vi "QD Load Debug Snapshot.vi"(6 "Variant in":variant, 7 "Shift Pressed?":bool, 8 "error in (no error)":errorcluster, 10 "QD Combo Box Ref":refnum<vi>, 11 "QD Launch VI Ref":refnum<vi>) -> (0 "error out":errorcluster, 4 "Variant out":variant)   [LabVIEW 2020]
doc: "Restore <b>Debug Snapshot</b> for the current VI. Use SHIFT to ignore breakpoints.\n\nDefault Shortcut - [l]"
uses:
  Public API.lvlib
  Type Definitions/Snapshot Handling Options--cluster.ctl
  Path Getter/Path Getter.lvclass
  C:/Users/juanj/Documents/hasbun_wood_engineering/github/Debug-Snapshots-for-LabVIEW/src/Path Getter/Path Getter.lvclass
  C:/Users/juanj/Documents/hasbun_wood_engineering/github/Debug-Snapshots-for-LabVIEW/src/IPath Getter/IPath Getter.lvclass
panel:
  in  "Undo Name":string="Quick Drop Keyboard Shortcut"
  # "Do not change the connector pane of this VI.\n\nSee the block diagram for directions on how to use this template."
  # "Specify the name of the Undo transaction"
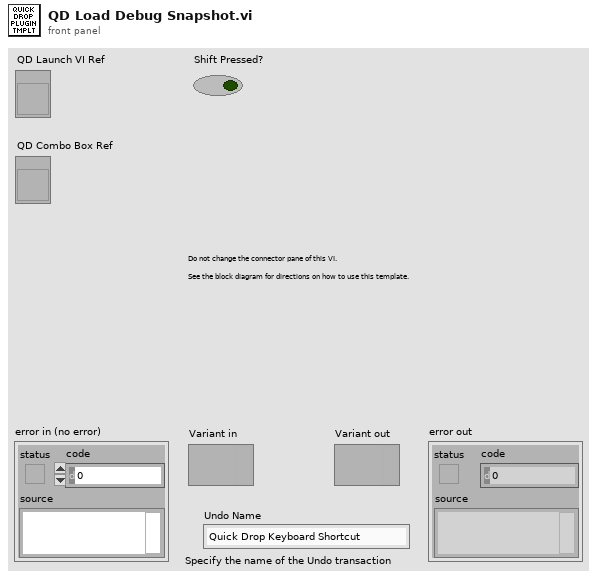
[diagram p1: front panel]
types:
  T1 = typedef "Snapshot Handling Options--cluster.ctl" = cluster{"Breakpoints":bool, "Probes":bool}
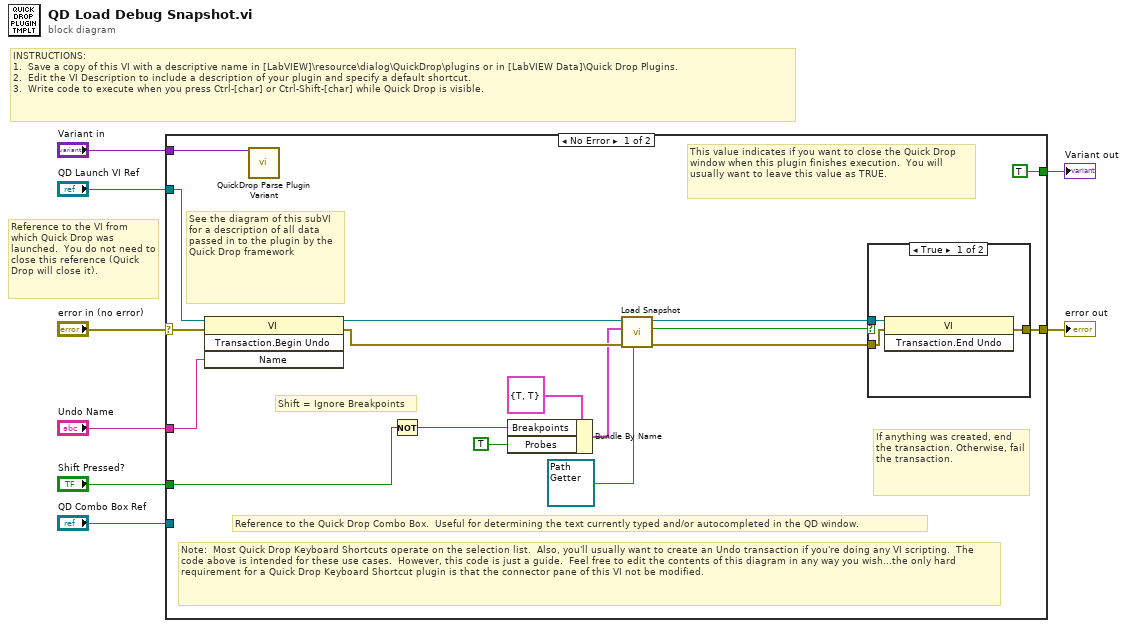
[diagram p0: block diagram]
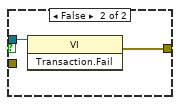
[diagram p2: hidden frame]
diagram:
  # "Reference to the VI from which Quick Drop was launched.  You do not need to close this reference (Quick Drop will close it)."
  # "INSTRUCTIONS:\n1.  Save a copy of this VI with a descriptive name in [LabVIEW]\\resource\\dialog\\QuickDrop\\plugins or in [LabVIEW Data]\\Quick Drop Plugins.\n2.  Edit the VI Description to include a description of your plugin and specify a default shortcut. \n3.  Write code to execute when you press Ctrl-[char] or Ctrl-Shift-[char] while Quick Drop is visible."
  n1 = case shown="No Error" "error in (no error)" {
    selector: "error in (no error)" -> [w24 w31]
    tunnel: [w20 w31] -> w7
    tunnel: "QD Launch VI Ref" -> [w23 _]
    tunnel: "Shift Pressed?" -> [w11 _]
    tunnel: "QD Combo Box Ref" -> [_ _]
    tunnel: "Variant in" -> [w25 _]
    tunnel: "Undo Name" -> [w22 _]
    tunnel: [TRUE _] -> w1
    frame No Error {
      # "Shift = Ignore Breakpoints"
      # "Note:  Most Quick Drop Keyboard Shortcuts operate on the selection list.  Also, you'll usually want to create an Undo transaction if you're doing any VI scripting.  The code above is intended for these use cases.  However, this code is just a guide.  Feel free to edit the contents of this diagram in any way you wish...the only hard requirement for a Quick Drop Keyboard Shortcut plugin is that the connector pane of this VI not be modified."
      # "If anything was created, end the transaction. Otherwise, fail the transaction."
      # "This value indicates if you want to close the Quick Drop window when this plugin finishes execution.  You will usually want to leave this value as TRUE."
      # "See the diagram of this subVI for a description of all data passed in to the plugin by the Quick Drop framework"
      # "Reference to the Quick Drop Combo Box.  Useful for determining the text currently typed and/or autocompleted in the QD window."
      n2 = invoke class="VI" method="Transaction.Begin Undo"(reference=w23, error in=w24, "Name"=w22) -> (reference out=w19:refnum<vi>, error out=w18:errorcluster)  [unwired: 1 in, 2 out]
      n3 = call <vilib>:"QuickDrop Parse Plugin Variant.vi"("QDKS Variant in"=w25) -> ()  [unwired: 12 in, 3 out]
      n4 = Not(x=w11) -> (.not. x?=w10:bool)
      n5 = Bundle By Name(cluster=T1 {"Breakpoints"=TRUE, "Probes"=TRUE} ("Debug Elements Options"), "Breakpoints"=w10, "Probes"=TRUE) -> (w15:T1)
      n6 = call "Load Snapshot.vi"("IPath Getter in"=refnum<class "Path Getter.lvclass"> refnum ("Path Getter.lvclass"), "error in"=w18, "Debug Elements Options"=w15, "VI Reference in"=w19) -> ("error out"=w12:errorcluster, "VI Modified"=w14:bool, "VI Reference out"=w13:refnum<vi>)  [unwired: 5 in]
      n7 = case shown="True" w14 {
        tunnel: w13 -> [w27 w29]
        tunnel: [w28 w30] -> w20
        tunnel: w12 -> [w26 _]
        frame True {
          n8 = invoke class="VI" method="Transaction.End Undo"(reference=w27, error in=w26) -> (error out=w28:errorcluster)  [unwired: 1 in, 2 out]
        }
        frame False {
          n9 = invoke class="VI" method="Transaction.Fail"(reference=w29) -> (error out=w30:errorcluster)  [unwired: 2 in, 2 out]
        }
      }
    }
    frame Error {
    }
  }
  "error out" <- w7
  "Variant out" <- w1
